vi "Stepper_Control.vi"() -> ()   [LabVIEW 2018]
uses:
  <vilib>/MakerHub/LINX/Public/Peripherals/Digital/Digital Write N Chans.vi
  <vilib>/MakerHub/LINX/Private/Local IO/LinxDigitalWrite.vi
  <vilib>/MakerHub/LINX/Public/Utilities/Check Channel.vi
  <vilib>/MakerHub/LINX/Public/Utilities/Open Serial.vi
  <vilib>/MakerHub/LINX/Private/Utilties/Generate Error.vi
  <vilib>/MakerHub/LINX/LMH-LINX.lvlib
panel:
  in  "Horizontal Pointer Slide":u32(slide) max=100 step=10 scale=0.0..100.0
  in  "stop":bool
  in  "RUN CCW":bool
  in  "RUN CW":bool
  in  "CCW":bool
  in  "CW":bool
  in  "Serial Port":refnum<visa-resource-name>="N/A"
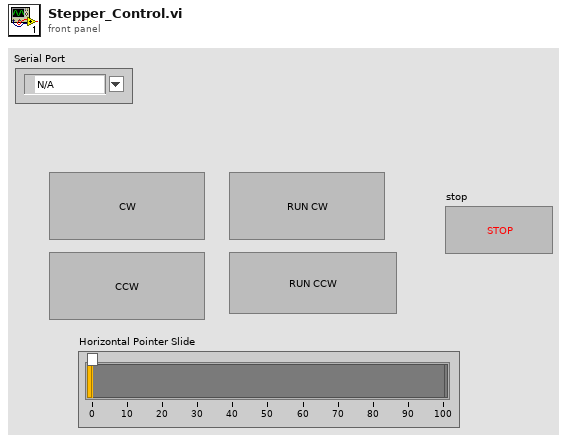
[diagram p1: front panel]
types:
  T1 = typedef "LMH-LINX.lvlib/LINX Ref.ctl" = cluster{"IO":T2, "Interface":T3, "LINX Device Config":T4}
  T2 = typedef "LMH-LINX.lvlib/Platform.ctl" = enum16{"Remote", "Local"}
  T3 = typedef "LMH-LINX.lvlib/Interface.ctl" = enum16{"Serial", "TCP"}
  T4 = typedef "LMH-LINX.lvlib/Device.lvlib/LINX Device Config.ctl" = cluster{"Interface":T3, "COM Port":refnum<visa-resource-name>, "TCP Configuration":T5, "Device Family":u8, "Device ID":u8, "Device Name":string, "TCP Ref":refnum<k5>, "Channels":T6}
  T5 = typedef "LMH-LINX.lvlib/Device.lvlib/TCP Config.ctl" = cluster{"IP Address":string, "Port":u16}
  T6 = typedef "LMH-LINX.lvlib/Channels.ctl" = cluster{"DI":u8[], "DO":u8[], "AI":u8[], "AO":u8[], "PWM":u8[], "QE":u8[], "UART":u8[], "I2C 2":u8[], "SPI":u8[], "CAN":u8[], "Servo":u8[], "AI Ref (V)":dbl, "AI Resolution (Bits)":u8, "AO Ref (V)":dbl, "AO Resolution (Bits)":u8}
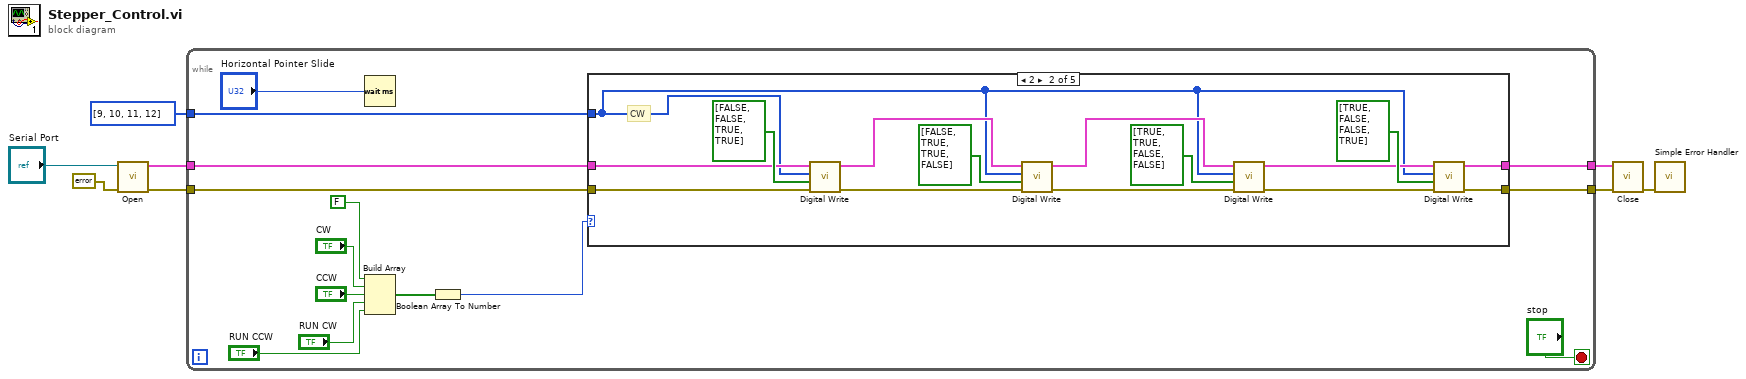
[diagram p0: block diagram]
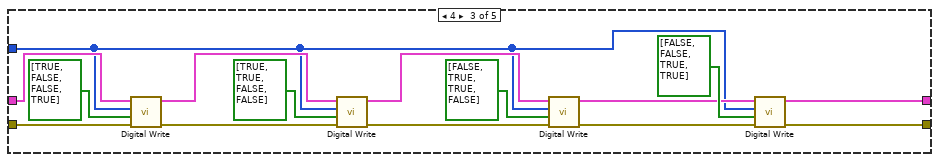
[diagram p3: hidden frame]
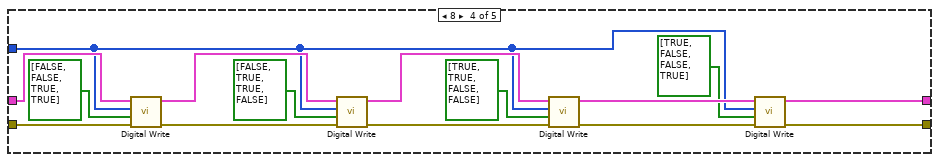
[diagram p4: hidden frame]
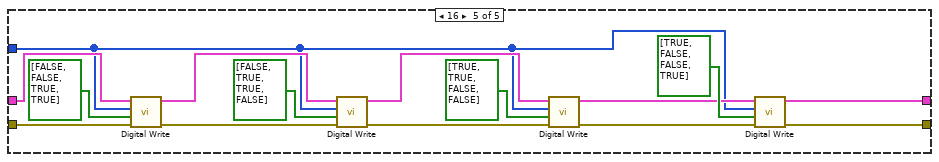
[diagram p5: hidden frame]
diagram:
  n1 = call-poly <vilib>:"Open.vi"("Error In"=errorcluster {"status"=FALSE, "code"=0, "source"=""}, "Serial Port"="Serial Port") -> ("Error Out"=w6:errorcluster, "LINX Resource"=w7:T1)  [unwired: 7 in, 1 out]
  n2 = while {
    tunnel: w7 -> [w15]
    tunnel: [w14] -> w5
    tunnel: w6 -> [w13]
    tunnel: [w12] -> w4
    tunnel: u8[] [9, 10, 11, 12] ("DO Channels") -> [w11]
    stop <- "stop" stop-if-true
    n3 = Wait (ms)(milliseconds to wait="Horizontal Pointer Slide") -> ()  [unwired: 1 out]
    n4 = Build Array "Build Array"(FALSE, "CW", "CCW", "RUN CW", "RUN CCW") -> (w17:bool[])
    n5 = Boolean Array To Number(Boolean array=w17) -> (number=w16:u32)
    n6 = case shown="2" w16 {
      tunnel: w15 -> [w23 w31 w43 w58 w73]
      tunnel: [w23 w27 w41 w56 w71] -> w14
      tunnel: w13 -> [w24 w36 w44 w59 w74]
      tunnel: [w24 w32 w40 w55 w70] -> w12
      tunnel: w11 -> [_ w26 w42 w57 w72]
      frame 0, Default {
      }
      frame 2 {
        # "CW"
        n7 = call-poly <vilib>:"Digital Write.vi"("Error In"=w36, "Values"=bool[] [FALSE, FALSE, TRUE, TRUE], "DO Channels"=w26, "LINX Resource"=w31) -> ("Error Out"=w35:errorcluster, "LINX Resource"=w30:T1)  [unwired: 6 in]
        n8 = call-poly <vilib>:"Digital Write.vi"("Error In"=w35, "Values"=bool[] [FALSE, TRUE, TRUE, FALSE], "DO Channels"=w26, "LINX Resource"=w30) -> ("Error Out"=w34:errorcluster, "LINX Resource"=w29:T1)  [unwired: 6 in]
        n9 = call-poly <vilib>:"Digital Write.vi"("Error In"=w34, "Values"=bool[] [TRUE, TRUE, FALSE, FALSE], "DO Channels"=w26, "LINX Resource"=w29) -> ("Error Out"=w33:errorcluster, "LINX Resource"=w28:T1)  [unwired: 6 in]
        n10 = call-poly <vilib>:"Digital Write.vi"("Error In"=w33, "Values"=bool[] [TRUE, FALSE, FALSE, TRUE], "DO Channels"=w26, "LINX Resource"=w28) -> ("Error Out"=w32:errorcluster, "LINX Resource"=w27:T1)  [unwired: 6 in]
      }
      frame 4 {
        n11 = call-poly <vilib>:"Digital Write.vi"("Error In"=w44, "Values"=bool[] [TRUE, FALSE, FALSE, TRUE], "DO Channels"=w42, "LINX Resource"=w43) -> ("Error Out"=w51:errorcluster, "LINX Resource"=w48:T1)  [unwired: 6 in]
        n12 = call-poly <vilib>:"Digital Write.vi"("Error In"=w51, "Values"=bool[] [TRUE, TRUE, FALSE, FALSE], "DO Channels"=w42, "LINX Resource"=w48) -> ("Error Out"=w50:errorcluster, "LINX Resource"=w47:T1)  [unwired: 6 in]
        n13 = call-poly <vilib>:"Digital Write.vi"("Error In"=w50, "Values"=bool[] [FALSE, TRUE, TRUE, FALSE], "DO Channels"=w42, "LINX Resource"=w47) -> ("Error Out"=w49:errorcluster, "LINX Resource"=w46:T1)  [unwired: 6 in]
        n14 = call-poly <vilib>:"Digital Write.vi"("Error In"=w49, "Values"=bool[] [FALSE, FALSE, TRUE, TRUE], "DO Channels"=w42, "LINX Resource"=w46) -> ("Error Out"=w40:errorcluster, "LINX Resource"=w41:T1)  [unwired: 6 in]
      }
      frame 8 {
        n15 = call-poly <vilib>:"Digital Write.vi"("Error In"=w59, "Values"=bool[] [FALSE, FALSE, TRUE, TRUE], "DO Channels"=w57, "LINX Resource"=w58) -> ("Error Out"=w64:errorcluster, "LINX Resource"=w67:T1)  [unwired: 6 in]
        n16 = call-poly <vilib>:"Digital Write.vi"("Error In"=w64, "Values"=bool[] [FALSE, TRUE, TRUE, FALSE], "DO Channels"=w57, "LINX Resource"=w67) -> ("Error Out"=w65:errorcluster, "LINX Resource"=w68:T1)  [unwired: 6 in]
        n17 = call-poly <vilib>:"Digital Write.vi"("Error In"=w65, "Values"=bool[] [TRUE, TRUE, FALSE, FALSE], "DO Channels"=w57, "LINX Resource"=w68) -> ("Error Out"=w66:errorcluster, "LINX Resource"=w69:T1)  [unwired: 6 in]
        n18 = call-poly <vilib>:"Digital Write.vi"("Error In"=w66, "Values"=bool[] [TRUE, FALSE, FALSE, TRUE], "DO Channels"=w57, "LINX Resource"=w69) -> ("Error Out"=w55:errorcluster, "LINX Resource"=w56:T1)  [unwired: 6 in]
      }
      frame 16 {
        n19 = call-poly <vilib>:"Digital Write.vi"("Error In"=w74, "Values"=bool[] [FALSE, FALSE, TRUE, TRUE], "DO Channels"=w72, "LINX Resource"=w73) -> ("Error Out"=w81:errorcluster, "LINX Resource"=w78:T1)  [unwired: 6 in]
        n20 = call-poly <vilib>:"Digital Write.vi"("Error In"=w81, "Values"=bool[] [FALSE, TRUE, TRUE, FALSE], "DO Channels"=w72, "LINX Resource"=w78) -> ("Error Out"=w80:errorcluster, "LINX Resource"=w77:T1)  [unwired: 6 in]
        n21 = call-poly <vilib>:"Digital Write.vi"("Error In"=w80, "Values"=bool[] [TRUE, TRUE, FALSE, FALSE], "DO Channels"=w72, "LINX Resource"=w77) -> ("Error Out"=w79:errorcluster, "LINX Resource"=w76:T1)  [unwired: 6 in]
        n22 = call-poly <vilib>:"Digital Write.vi"("Error In"=w79, "Values"=bool[] [TRUE, FALSE, FALSE, TRUE], "DO Channels"=w72, "LINX Resource"=w76) -> ("Error Out"=w70:errorcluster, "LINX Resource"=w71:T1)  [unwired: 6 in]
      }
    }
  }
  n23 = call <vilib>:"Close.vi"("Error In"=w4, "LINX Resource"=w5) -> ("Error Out"=w3:errorcluster)  [unwired: 9 in]
  n24 = call <vilib>:"Simple Error Handler.vi"("error in (no error)"=w3) -> ()  [unwired: 4 in, 5 out]
